vi "NXT SetSpeed.vi"(4 "error in (no error)":errorcluster, 6 "Speed":u8=5) -> (0 "error out":errorcluster)   [LabVIEW 2012]
uses:
  <vilib>/NXT/NXT Controls/NXTInputRefnum.ctl
  <vilib>/NXT/NXT Controls/NXTSyscallRefnum.ctl
  <resource>/objmgr/NXTInputOutput.rc
panel:
  in  "Sys Call Refnum":T1
  in  "Sensor Refnum":T2
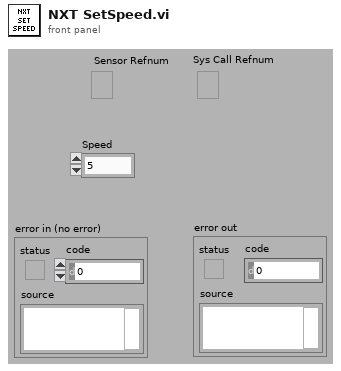
[diagram p1: front panel]
types:
  T1 = typedef "NXTSyscallRefnum.ctl" = refnum<k21>
  T2 = typedef "NXTInputRefnum.ctl" = refnum<k21>
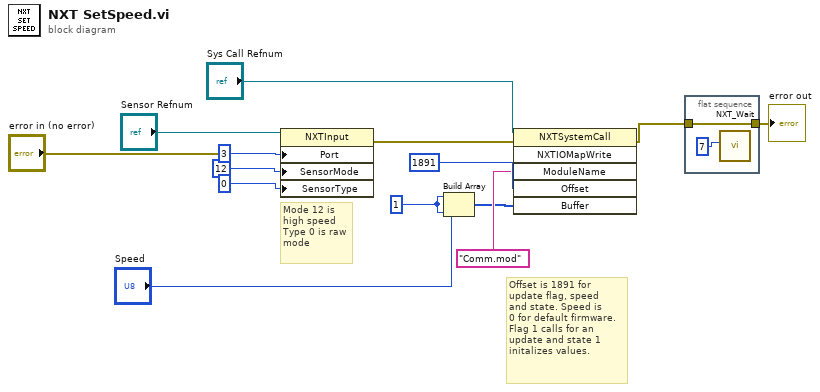
[diagram p0: block diagram]
diagram:
  w4 = u8 1 ("Offset")
  # "Offset is 1891 for\nupdate flag, speed\nand state. Speed is \n0 for default firmware.\nFlag 1 calls for an \nupdate and state 1 \ninitalizes values."
  # "Mode 12 is\nhigh speed\nType 0 is raw\nmode"
  n1 = property class="NXTInput"(reference="Sensor Refnum", error in="error in (no error)", "Port"=u8 3, "SensorMode"=u8 12, "SensorType"=u8 0) -> (error out=w10:errorcluster)  [unwired: 1 out]
  n2 = Build Array(w4, "Speed", w4) -> (w5:u8[])
  n3 = invoke class="NXTSystemCall" method="NXTIOMapWrite"(reference="Sys Call Refnum", error in=w10, "ModuleName"="Comm.mod", "Offset"=u16 1891, "Buffer"=w5) -> (error out=w6:errorcluster)  [unwired: 1 in, 5 out]
  n4 = flat-sequence {
    tunnel: w6 -> [w15]
    tunnel: [w15] -> w2
    frame #0 {
      n5 = call <vilib>:"NXT_Wait.vi"("Wait (ms)"=u32 7) -> ()  [unwired: 9 in, 2 out]
    }
  }
  "error out" <- w2
